vi "Matrix Condition Number.vi"   [LabVIEW 2018, in "NI_AALPro.lvlib"]
doc: "Computes the <B>condition number</B> of <B>Input Matrix</B>. Wire data to the <B>Input Matrix</B> input to determine the polymorphic instance to use or manually select the instance."
uses:
  <vilib>/Analysis/NI_AALPro.lvlib
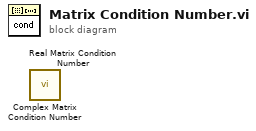
[diagram p0: block diagram]
diagram:
  n1 = call "Complex Matrix Condition Number.vi"() -> ()  [unwired: 2 in, 2 out]
  n2 = call "Real Matrix Condition Number.vi"() -> ()  [unwired: 2 in, 2 out]
